vi "PH_BL-Master.PC _getO2DevStatus.vi"(0 "i ref in":refnum<vi>, 2 "O2 Instance":string, 3 "Status":T1 items=["no info", "off/false/out", "on/true/in", "Failure", "Alarm", "Status 1", "Status 2", "Status 3"], 5 "error in (no error)":errorcluster) -> (14 "i ref out":refnum<vi>, 19 "error out":errorcluster)   [LabVIEW 2014, in "PH_BL-Master.lvlib"]
doc: "This VI writes the incoming information to own attributes."
uses:
  PH_BL-Master.lvlib
  PH_StatusHandler/PH_StatusHandler.Status.ctl
  PH_StatusHandler/PH_StatusHandler.lvlib
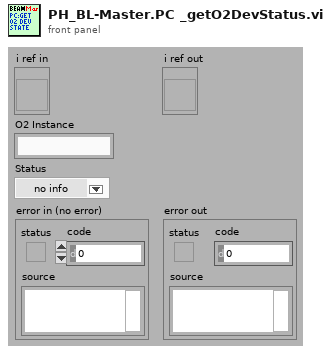
[diagram p1: front panel]
types:
  T1 = typedef "PH_StatusHandler.lvlib/PH_StatusHandler.Status.ctl" = i16
  T2 = typedef "PH_BL-Master.lvlib/PH_BL-Master.i attribute.ctl" = cluster{"Remote controlled":bool, "Boolean Condition Service Subscriber":refnum<vi>[], "Picture Condition Service Subscriber":refnum<vi>[], "R2S":cluster{"GUI Ref":refnum<vi>, "State":bool}, "Vacua":cluster{"GUI Ref":refnum<vi>, "Limit":dbl, "Curr Value":dbl, "in range":bool}[], "O2 Inspection":cluster{"GUI Ref":refnum<vi>, "Concentration":dbl, "State":T1}[], "Boolean Status Service Subscriber":cluster{"GUI Ref":refnum<vi>, "Status":T1, "no Link?":bool, "Status Subscriber Class":T3}[], "Picture Status Service Subscriber":cluster{"GUI Ref":refnum<vi>, "Status":T1, "no Link?":bool, "Status Subscriber Class":T3}[], "6P 4Q Service Subscriber":cluster{"GUI Ref":refnum<vi>, "Selector":T4, "no Link?":bool}[], "Index of latest 6P 4Q changing Instance":i32, "Index of latest Picture Status changing Instance":i32, "Index of latest Boolean Status changing Instance":i32, "Vision ID on same Node":string, "Start Phase over?":bool, "GUI Ref Delete":refnum<vi>}
  T3 = typedef "PH_BL-Master.lvlib/PH_BL-Master.Status Subscriber Class.ctl" = enum16{"unknown", "Switch", "BB", "6P Switch", "Switch GUI", "Switch and 6P State", "Force Sensor"}
  T4 = typedef "PH_4_Pos_Selector.lvlib/PH_4_Pos_Selector.Position Selector.ctl" = u16
  T5 = cluster{"GUI Ref":refnum<vi>, "Concentration":dbl, "State":T1}[]
  T6 = cluster{"GUI Ref":refnum<vi>, "Concentration":dbl, "State":T1}
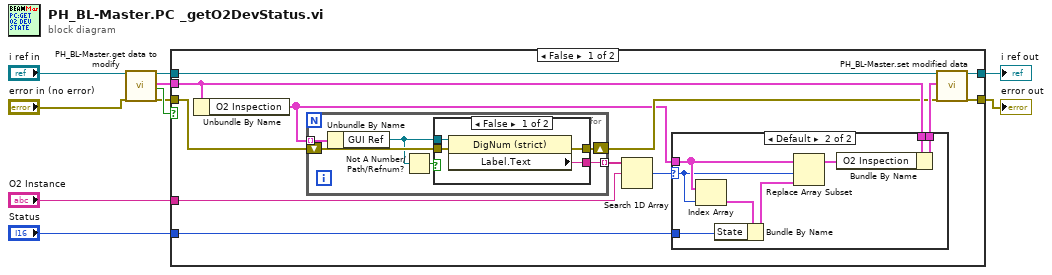
[diagram p0: block diagram]
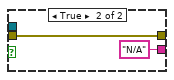
[diagram p3: hidden frame]
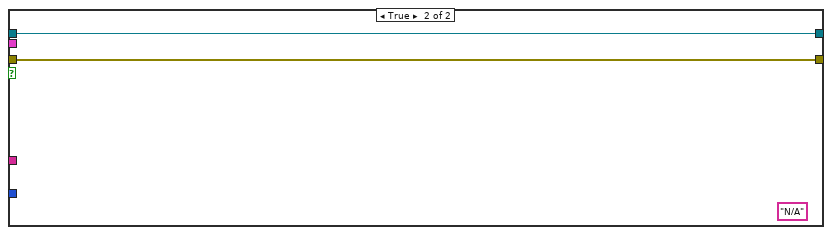
[diagram p4: hidden frame]
diagram:
  n1 = call "PH_BL-Master.get data to modify.vi"("i ref in"="i ref in", "error in (no error)"="error in (no error)") -> ("i ref out"=w5:refnum<vi>, "i attribute"=w9:T2, "timed out"=w10:bool, "error out"=w7:errorcluster)  [unwired: 14 in]
  n2 = case shown="False" w10 {
    tunnel: w5 -> [w20 w45]
    tunnel: [w22 w45] -> w6
    tunnel: w7 -> [w16 w44]
    tunnel: [w21 w44] -> w8
    tunnel: w9 -> [w18 _]
    tunnel: "Status" -> [w13 _]
    tunnel: "O2 Instance" -> [w11 _]
    frame False {
      n3 = Unbundle By Name(w18) -> ("O2 Inspection"=w12:T5)
      n4 = for {
        tunnel: w12 -> [w33] mode=indexing
        tunnel: [w37] -> w17 mode=indexing
        shift-right: [w35] -> w14
        shift-left: w16 -> [w36]
        n5 = Unbundle By Name(w33) -> ("GUI Ref"=w32:refnum<vi>)
        n6 = Not A Number/Path/Refnum?(number/path/refnum=w32) -> (NaN/Path/Refnum?=w34:bool)
        n7 = case shown="False" w34 {
          tunnel: w32 -> [w41 _]
          tunnel: [w40 "N/A" ("Label.Text")] -> w37
          tunnel: w36 -> [w39 w43]
          tunnel: [w38 w43] -> w35
          frame False {
            n8 = property class="DigNum (strict)"(reference=w41, error in=w39) -> (error out=w38:errorcluster, "Label.Text"=w40:string)  [unwired: 1 out]
          }
          frame True {
          }
        }
      }
      n9 = Search 1D Array(1D array=w17, element=w11) -> (index of element=w15:i32)  [unwired: 1 in]
      n10 = case shown="Default" w15 {
        selector: w15 -> [_ w27]
        tunnel: [w23 w31] -> w19
        tunnel: w18 -> [w23 w30]
        tunnel: w12 -> [_ w28]
        tunnel: w13 -> [_ w25]
        frame -1 {
        }
        frame Default {
          n11 = Index Array(array=w28, index=w27) -> (element=w26:T6)
          n12 = Bundle By Name(cluster=w26, "State"=w25) -> (w24:T6)
          n13 = Replace Array Subset(array=w28, new element=w24, index=w27) -> (w29:T5)
          n14 = Bundle By Name(cluster=w30, "O2 Inspection"=w29) -> (w31:T2)
        }
      }
      n15 = call "PH_BL-Master.set modified data.vi"("i ref in"=w20, "i attribute"=w19, "error in (no error)"=w14) -> ("i ref out"=w22:refnum<vi>, "error out"=w21:errorcluster)  [unwired: 15 in]
    }
    frame True {
      (unwired) "N/A" ("Service Name")
    }
  }
  "error out" <- w8
  "i ref out" <- w6
